vi "CRYIR For TSR.vi"(6 "EQ information":T2={"Stimulus EQ Curve"={"Name"="", "Curve"=[], "X data"=1, "Y data"=1, "Z data"=1, "X axis"=0, "Y axis"=1, "Z axis"=1, "X unit"="Hz", "Y unit"="", "Z unit"="deg.", "X dB ref"=1.0, "Y dB ref"=1.0, "Z dB ref"=1.0, "single val"=FALSE, "protected"=FALSE, "display X"=TRUE, "display Y"=TRUE, "display Z"=TRUE, "Test Info"="", "Step No."=0, "Plot Settings"={"Color"=0, "Interpolation"=0, "Point Style"=0, "Line Style"=0, "Point Color"=0, "Line Width"=0, "Bar Plot Style"=0, "Fill To"=0}, "AutoProtect"=FALSE}, "EQ"=FALSE, "EQ Rate"=0.0} {"EQ Rate" format="%.2f"; "Stimulus EQ Curve"."Z data" items=["dB", "Lin"]; "Stimulus EQ Curve"."X data" items=["dB", "Lin"]; "Stimulus EQ Curve"."Y data" items=["dB", "Lin"]; "Stimulus EQ Curve"."Z dB ref" format="%.1f"; "Stimulus EQ Curve"."Z axis" items=["Log", "Lin"]; "Stimulus EQ Curve"."X dB ref" format="%.1f"; "Stimulus EQ Curve"."X axis" items=["Log", "Lin"]; "Stimulus EQ Curve"."Y axis" items=["Log", "Lin"]; "Stimulus EQ Curve"."Y dB ref" format="%.1f"; "Stimulus EQ Curve"."Curve"."z" format="%.2f"; "Stimulus EQ Curve"."Curve"."y" format="%.2f"; "Stimulus EQ Curve"."Curve"."x" format="%.2f"}, 8 "Fs":dbl=44100.0, 9 "Abs/Rel":u16(ring) items=["Absolute", "Relative"], 10 "Response[y(t)]":dbl[](array[numeric]) format="%.2f", 11 "Stimulus[x(t)]":dbl[](array[numeric]) format="%.2f") -> (0 "T0":dbl, 1 "T max Index":dbl, 2 "T max Amplitude":dbl, 3 "Deconvolved Response":cdb[](array[numeric]) format="%.2f", 4 "T max Time":dbl)   [LabVIEW 2013]
uses:
  Typedef Control/CRYData Cluster.ctl
  <vilib>/Analysis/2dsp.llb/Real FFT.vi
  <vilib>/Analysis/NI_AALPro.lvlib
panel:
  out "Impulse Wave graph":cluster{"t0S":dbl, dbl, "timeHistory":dbl[]}(graph)
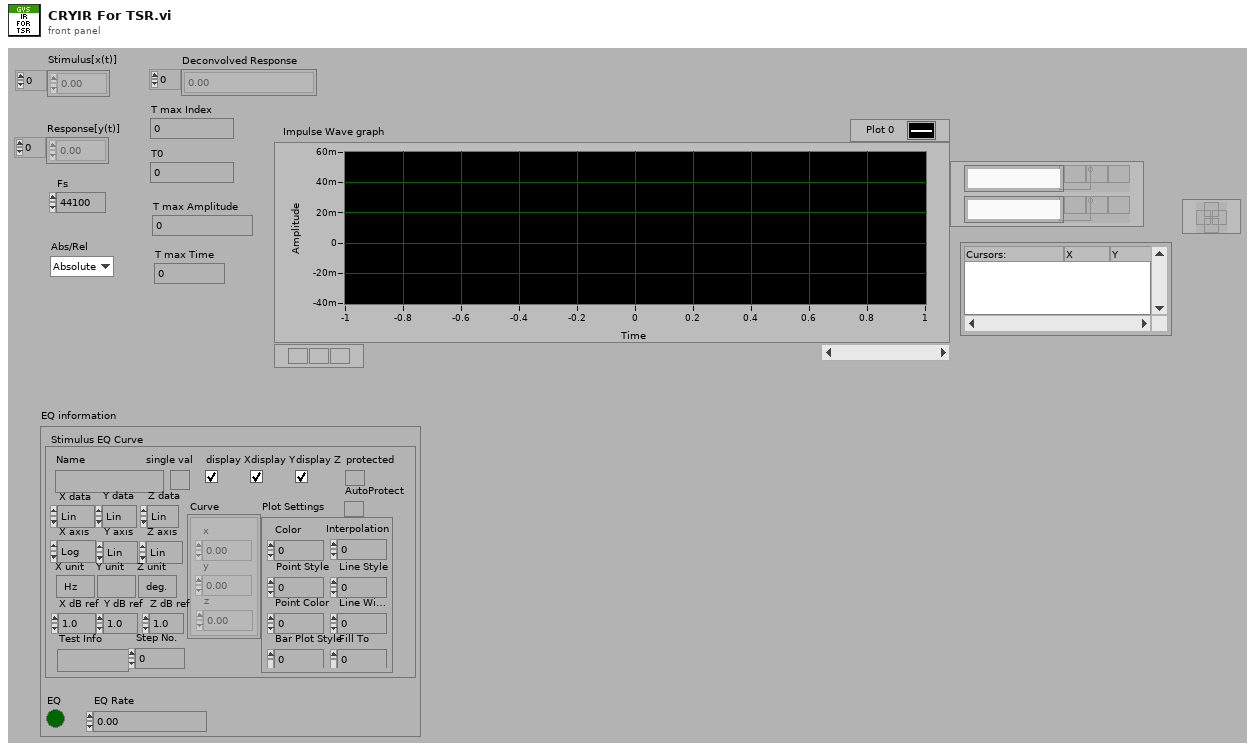
[diagram p1: front panel]
types:
  T1 = typedef "CRYData Cluster.ctl" = cluster{"Name":string, "Curve":cluster{"x":dbl, "y":dbl, "z":dbl}[], "X data":u16, "Y data":u16, "Z data":u16, "X axis":u16, "Y axis":u16, "Z axis":u16, "X unit":string, "Y unit":string, "Z unit":string, "X dB ref":dbl, "Y dB ref":dbl, "Z dB ref":dbl, "single val":bool, "protected":bool, "display X":bool, "display Y":bool, "display Z":bool, "Test Info":string, "Step No.":i32, "Plot Settings":cluster{"Color":u32, "Interpolation":u8, "Point Style":u8, "Line Style":u8, "Point Color":u32, "Line Width":u8, "Bar Plot Style":u8, "Fill To":i16}, "AutoProtect":bool}
  T2 = cluster{"Stimulus EQ Curve":T1, "EQ":bool, "EQ Rate":dbl}
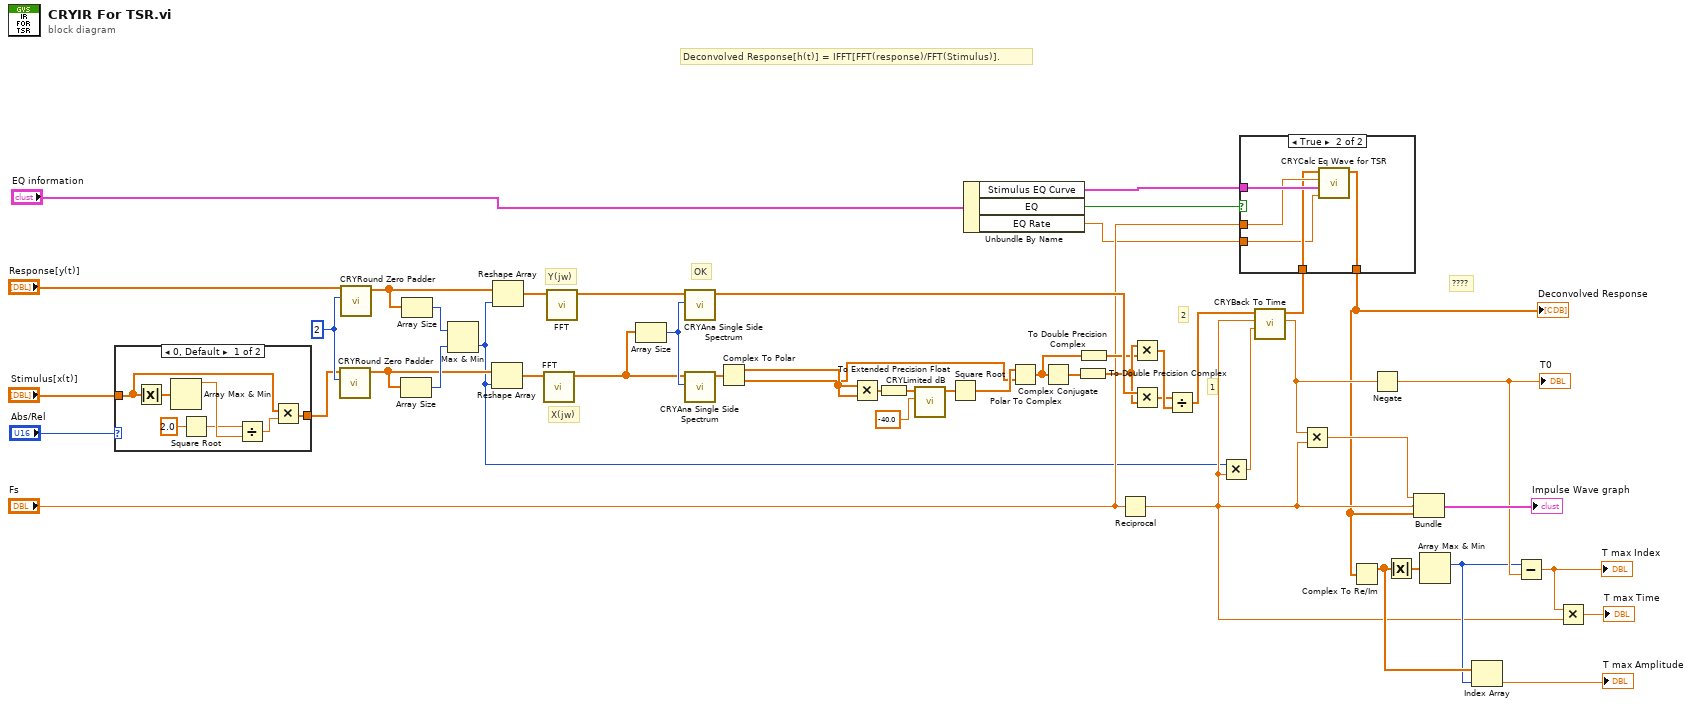
[diagram p0: block diagram]
diagram:
  w47 = u8 2 ("Significant Digit")
  # "????"
  # "2"
  # "1"
  # "OK"
  # "X(jw)"
  # "Y(jw)"
  # "Deconvolved Response[h(t)] = IFFT[FFT(response)/FFT(Stimulus)]."
  n1 = case shown="0, Default" "Abs/Rel" {
    tunnel: [w56 w58] -> w6
    tunnel: "Stimulus[x(t)]" -> [w55 w58]
    frame 0, Default {
      n2 = Absolute Value(x=w55) -> (abs(x)=w54:dbl[])
      n3 = Array Max & Min(array=w54) -> (max value=w53:dbl)  [unwired: 3 out]
      n4 = Square Root(x=2.0) -> (sqrt(x)=w51:dbl)
      n5 = Divide(x=w51, y=w53) -> (x/y=w52:dbl)
      n6 = Multiply(x=w55, y=w52) -> (x*y=w56:dbl[])
    }
    frame 1 {
    }
  }
  n7 = call "CRYRound Zero Padder.vi"("Significant Digit"=w47, "Vector in"=w6) -> ("Zero Padder Vector out"=w32:dbl[])  [unwired: 8 in, 1 out]
  n8 = call "CRYRound Zero Padder.vi"("Significant Digit"=w47, "Vector in"="Response[y(t)]") -> ("Zero Padder Vector out"=w31:dbl[])  [unwired: 8 in, 1 out]
  n9 = Array Size(array=w32) -> (size(s)=w48:i32)
  n10 = Array Size(array=w31) -> (size(s)=w49:i32)
  n11 = Max & Min(x=w49, y=w48) -> (min(x,y)=w1:i32)  [unwired: 1 out]
  n12 = Reshape Array(w32, w1) -> (w46:dbl[])
  n13 = Reshape Array(w31, w1) -> (w45:dbl[])
  n14 = call-poly <vilib>:"FFT.vi"("X"=w46) -> ("FFT {X}"=w3:cdb[])  [unwired: 2 in, 8 out]
  n15 = call-poly <vilib>:"FFT.vi"("X"=w45) -> ("FFT {X}"=w4:cdb[])  [unwired: 2 in, 8 out]
  n16 = Array Size(array=w3) -> (size(s)=w35:i32)
  n17 = call "CRYAna Single Side Spectrum.vi"("FFT Size"=w35, "FFT"=w4) -> ("Single FFT"=w26:cdb[])  [unwired: 8 in, 1 out]
  n18 = call "CRYAna Single Side Spectrum.vi"("FFT Size"=w35, "FFT"=w3) -> ("Single FFT"=w44:cdb[])  [unwired: 8 in, 1 out]
  n19 = Complex To Polar(r * e^(i*theta)=w44) -> (r=w38:dbl[], theta=w36:dbl[])
  n20 = Multiply(x=w38, y=w38) -> (x*y=w43:dbl[])
  n21 = To Extended Precision Float(1:w43) -> (0:w40:ext[])
  n22 = call "CRYLimited dB.vi"("Dynamic(dB)"=-40.0, "Power spectrum"=w40) -> ("Limited spectrum"=w39:ext[])  [unwired: 9 in]
  n23 = Square Root(x=w39) -> (sqrt(x)=w37:ext[])
  n24 = Unbundle By Name("EQ information") -> ("Stimulus EQ Curve"=w11:T1, "EQ"=w5:bool, "EQ Rate"=w2:dbl)
  n25 = Polar To Complex(1:w36, 2:w37) -> (0:w22:cxt[])
  n26 = Complex Conjugate(1:w22) -> (0:w24:cxt[])
  n27 = To Double Precision Complex(1:w24) -> (0:w23:cdb[])
  n28 = To Double Precision Complex(1:w22) -> (0:w21:cdb[])
  n29 = Reciprocal(x="Fs") -> (1/x=w14:dbl)
  n30 = Multiply(x=w23, y=w21) -> (x*y=w42:cdb[])
  n31 = Multiply(x=w26, y=w23) -> (x*y=w41:cdb[])
  n32 = Divide(x=w41, y=w42) -> (x/y=w30:cdb[])
  n33 = Multiply(x=w1, y=w14) -> (x*y=w29:dbl)
  n34 = call "CRYBack To Time.vi"("T(s)"=w29, "dt(s)"=w14, "Spectrum"=w30) -> ("t0S"=w20:dbl, "timeHistory"=w9:cdb[])  [unwired: 7 in]
  n35 = case shown="True" w5 {
    tunnel: w11 -> [_ w64]
    tunnel: "Fs" -> [_ w63]
    tunnel: w9 -> [w59 w62]
    tunnel: [w59 w61] -> w8
    tunnel: w2 -> [_ w60]
    frame False {
    }
    frame True {
      n36 = call "CRYCalc Eq Wave for TSR.vi"("EQ Rate"=w60, "EQ Curve"=w64, "Fs"=w63, "Wave In"=w62) -> ("Wave Out"=w61:dbl[])  [unwired: 6 in, 1 out]
    }
  }
  "Deconvolved Response" <- w8
  n37 = Multiply(x=w20, y=w14) -> (x*y=w19:dbl)
  n38 = Complex To Re/Im(x + iy=w8) -> (x=w18:dbl[])  [unwired: 1 out]
  n39 = Negate(x=w20) -> (-x=w28:dbl)
  "T0" <- w28
  n40 = Absolute Value(x=w18) -> (abs(x)=w27:dbl[])
  n41 = Bundle(w19, w14, "timeHistory"=w8) -> (→"Impulse Wave graph":cluster{dbl, dbl, "timeHistory":cdb[]})  [unwired: 1 in]
  n42 = Array Max & Min(array=w27) -> (max index (indices)=w17:i32)  [unwired: 3 out]
  n43 = Index Array(array=w18, index=w17) -> (element=→"T max Amplitude":dbl)
  n44 = Subtract(x=w17, y=w28) -> (x-y=w15:dbl)
  "T max Index" <- w15
  n45 = Multiply(x=w15, y=w14) -> (x*y=→"T max Time":dbl)
